vi "DatabaseUISpecificInfo.vi"(0 "UserBasicInfo":refnum<class "UserBasicInfo.lvclass">, 11 "error in (no error)":errorcluster) -> (4 "UserBasicInfo out":refnum<class "UserBasicInfo.lvclass">, 6 "TableName":string, 8 "BasicInfoTableColumn":string[](array[string]), 10 "column information":T1[](array[typedef])=[{"column name"="ID", "data type"=enum."Long (I32)", "size"=0, "allow null?"=FALSE}, {"column name"="姓名", "data type"=enum."String", "size"=0, "allow null?"=FALSE}, {"column name"="学院", "data type"=enum."String", "size"=0, "allow null?"=FALSE}, {"column name"="年级", "data type"=enum."String", "size"=0, "allow null?"=FALSE}, {"column name"="组别", "data type"=enum."String", "size"=0, "allow null?"=TRUE}, {"column name"="简介", "data type"=enum."String", "size"=0, "allow null?"=TRUE}], 15 "error out":errorcluster)   [LabVIEW 2015, in "UserManagement.lvlib" / "UserBasicInfo.lvclass"]
uses:
  UserManagement/UserBasicInfo/UserBasicInfo.lvclass
  <vilib>/addons/database/Auxilliary.llb/DB Tools Column Info.ctl
  <vilib>/addons/database/Auxilliary.llb/DB Tools DataTypes.ctl
  <vilib>/addons/database/NI_Database_API.lvlib
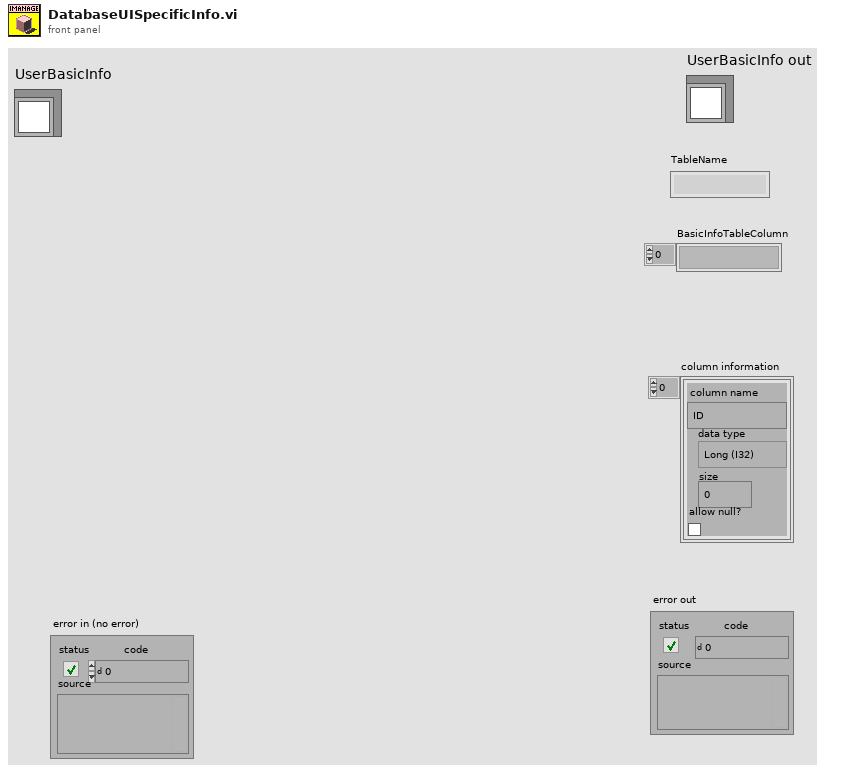
[diagram p1: front panel]
types:
  T1 = typedef "NI_Database_API.lvlib/DB Tools Column Info.ctl" = cluster{"column name":string, "data type":T2, "size":i32, "allow null?":bool}
  T2 = typedef "NI_Database_API.lvlib/DB Tools DataTypes.ctl" = enum16{"String", "Long (I32)", "Single (SGL)", "Double (DBL)", "Date/Time", "Binary"}
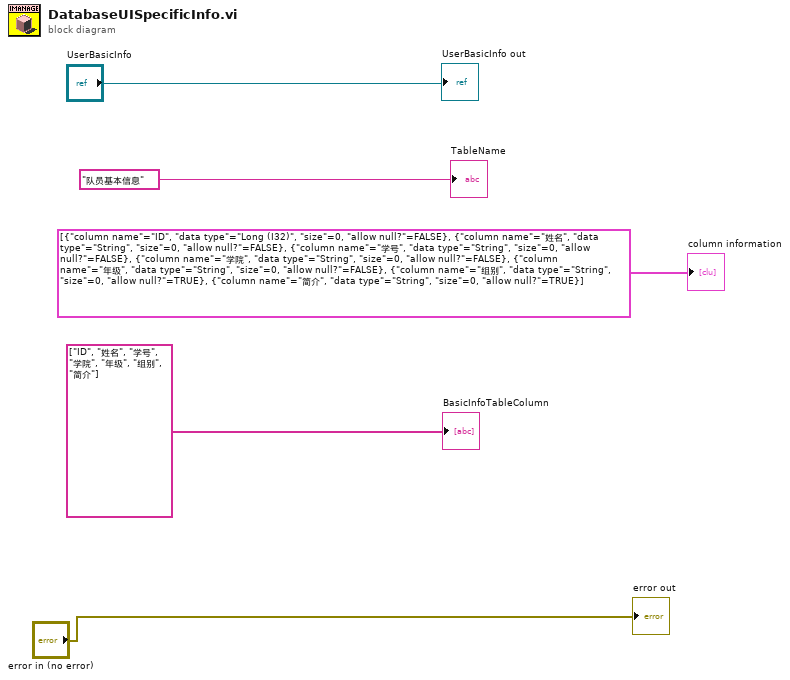
[diagram p0: block diagram]
diagram:
  "BasicInfoTableColumn" <- string[] ["ID", "姓名", "学号", "学院", "年级", "组别", "简介"]
  "TableName" <- "队员基本信息" ("TableName")
  "error out" <- "error in (no error)"
  "column information" <- T1[] [{"column name"="ID", "data type"=enum."Long (I32)", "size"=0, "allow null?"=FALSE}, {"column name"="姓名", "data type"=enum."String", "size"=0, "allow null?"=FALSE}, {"column name"="学号", "data type"=enum."String", "size"=0, "allow null?"=FALSE}, {"column name"="学院", "data type"=enum."String", "size"=0, "allow null?"=FALSE}, {"column name"="年级", "data type"=enum."String", "size"=0, "allow null?"=FALSE}, {"column name"="组别", "data type"=enum."String", "size"=0, "allow null?"=TRUE}, {"column name"="简介", "data type"=enum."String", "size"=0, "allow null?"=TRUE}] ("column information")
  "UserBasicInfo out" <- "UserBasicInfo"
